vi "Axes_settled.vi"(0 "System no.":i32=1 min=1 max=4 step=1, 2 "Conn. Axes":string[](array[string]), 3 "Settle window":dbl=0.01, 4 "Settle time/ms":u32=100, 5 "error in":errorcluster) -> (14 "Settled?":bool, 16 "Position":dbl[](array[numeric]) format="%.4f", 19 "error out":errorcluster)   [LabVIEW 2020]
doc: "Returns the axes settled state which is a software mapping of the ONT? firmware command. Positions must be within the settle window during the settle time to be settled. This VI can take up to the time specified by the Settle time control."
panel:
  # "Returns the settled state of the connected axes"
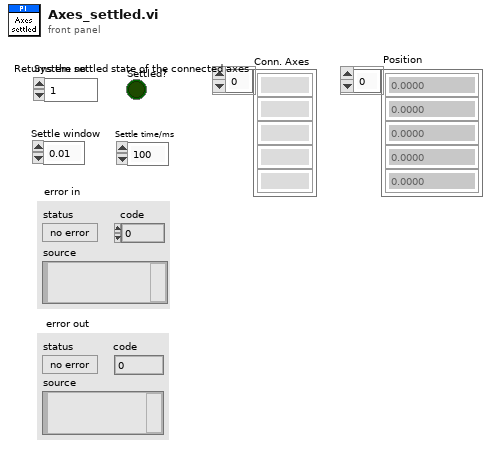
[diagram p1: front panel]
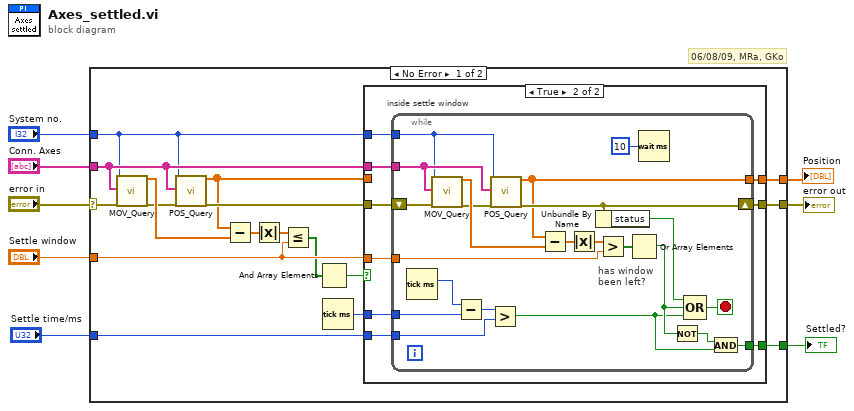
[diagram p0: block diagram]
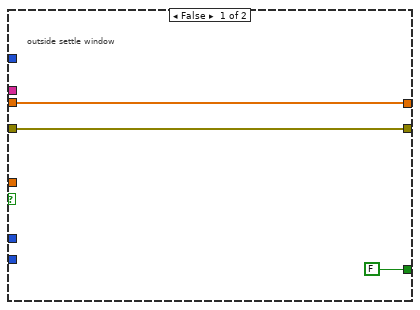
[diagram p2: hidden frame]
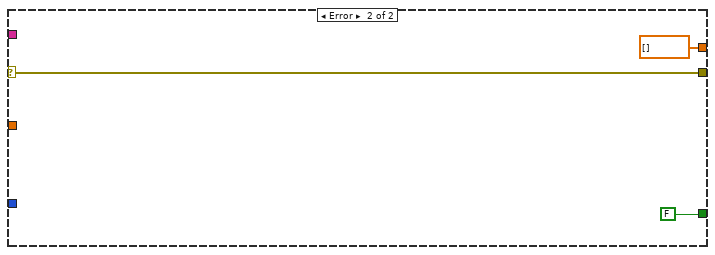
[diagram p3: hidden frame]
diagram:
  # "06/08/09, MRa, GKo"
  n1 = case shown="No Error" "error in" {
    selector: "error in" -> [w25 w62]
    tunnel: [w12 w62] -> w7
    tunnel: "Conn. Axes" -> [w17 _]
    tunnel: "Settle window" -> [w16 _]
    tunnel: "Settle time/ms" -> [w24 _]
    tunnel: "System no." -> [w14 _]
    tunnel: [w11 FALSE] -> w2
    tunnel: [w10 dbl[] [] ("Position")] -> w1
    frame No Error {
      n2 = call "MOV_Query.vi"("System no."=w14, "Axes to query"=w17, "error in"=w25) -> ("Target position"=w22:dbl[], "error out"=w21:errorcluster)  [unwired: 2 in, 13 out]
      n3 = call "POS_Query.vi"("System no."=w14, "Axes to query"=w17, "error in"=w21) -> ("Position"=w9:dbl[], "error out"=w18:errorcluster)  [unwired: 2 in, 13 out]
      n4 = Subtract(x=w9, y=w22) -> (x-y=w20:dbl[])
      n5 = Absolute Value(x=w20) -> (abs(x)=w23:dbl[])
      n6 = Less Or Equal?(x=w23, y=w16) -> (x <= y?=w13:bool[])
      n7 = And Array Elements(Boolean array=w13) -> (logical AND=w19:bool)
      n8 = Tick Count (ms)() -> (millisecond timer value=w15:u32)
      n9 = case shown="True" w19 {
        tunnel: w24 -> [_ w33]
        tunnel: w18 -> [w27 w37]
        tunnel: w17 -> [_ w36]
        tunnel: w16 -> [_ w35]
        tunnel: w15 -> [_ w34]
        tunnel: w14 -> [_ w32]
        tunnel: [FALSE w31] -> w11
        tunnel: [w27 w30] -> w12
        tunnel: [w26 w29] -> w10
        tunnel: w9 -> [w26 _]
        frame False {
          # "outside settle window"
        }
        frame True {
          # "inside settle window"
          n10 = while {
            shift-right: [w47] -> w30
            shift-left: w37 -> [w54]
            tunnel: w36 -> [w53]
            tunnel: w35 -> [w51]
            tunnel: w34 -> [w50]
            tunnel: w33 -> [w49]
            tunnel: w32 -> [w44]
            tunnel: [w39] -> w31
            tunnel: [w38] -> w29
            stop <- w43 stop-if-true
            # "has window\nbeen left?"
            n11 = Tick Count (ms)() -> (millisecond timer value=w59:u32)
            n12 = call "MOV_Query.vi"("System no."=w44, "Axes to query"=w53, "error in"=w54) -> ("Target position"=w57:dbl[], "error out"=w56:errorcluster)  [unwired: 2 in, 13 out]
            n13 = Subtract(x=w59, y=w50) -> (x-y=w48:u32)
            n14 = Greater?(x=w48, y=w49) -> (0:w41:bool)
            n15 = call "POS_Query.vi"("System no."=w44, "Axes to query"=w53, "error in"=w56) -> ("Position"=w38:dbl[], "error out"=w47:errorcluster)  [unwired: 2 in, 13 out]
            n16 = Subtract(x=w38, y=w57) -> (x-y=w55:dbl[])
            n17 = Absolute Value(x=w55) -> (abs(x)=w58:dbl[])
            n18 = Unbundle By Name(w47) -> ("status"=w46:bool)
            n19 = Greater?(x=w58, y=w51) -> (0:w52:bool[])
            n20 = Or Array Elements(Boolean array=w52) -> (logical OR=w42:bool)
            n21 = Wait (ms)(milliseconds to wait=u32 10) -> ()  [unwired: 1 out]
            n22 = Not(x=w42) -> (.not. x?=w40:bool)
            n23 = Compound Arithmetic op=OR(w46, w42, w41) -> (w43:bool)
            n24 = And(x=w40, y=w41) -> (x .and. y?=w39:bool)
          }
        }
      }
    }
    frame Error {
    }
  }
  "error out" <- w7
  "Settled?" <- w2
  "Position" <- w1
